vi "Transmitter.vi"() -> ()   [LabVIEW 2022 SP3]
uses:
  Transmitter States.ctl
  <vilib>/MakerHub/LINX/Public/Peripherals/Digital/Digital Write 1 Chan.vi
  <vilib>/MakerHub/LINX/Public/Peripherals/Digital/Digital Write N Chans.vi
  <vilib>/MakerHub/LINX/Private/Local IO/LinxDigitalWrite.vi
  <vilib>/MakerHub/LINX/Public/Utilities/Check Channel.vi
  <vilib>/MakerHub/LINX/Public/Utilities/Open Serial.vi
  <vilib>/MakerHub/LINX/Private/Utilties/Generate Error.vi
  <vilib>/MakerHub/LINX/LMH-LINX.lvlib
panel:
  out "Message Translated to Morse":string
  in  "stop":bool
  in  "Send Morse":bool
  in  "Message to Encode":string
  in  "Pulse Interval (ms)":u32=100
  in  "Serial Port":refnum<visa-resource-name>="N/A"
  in  "LED Channel":u8
  out "Message Transmitted":bool
  out "Digital Write Out":errorcluster
  out "File IO Error":errorcluster
  # "Morse Code Transmitter"
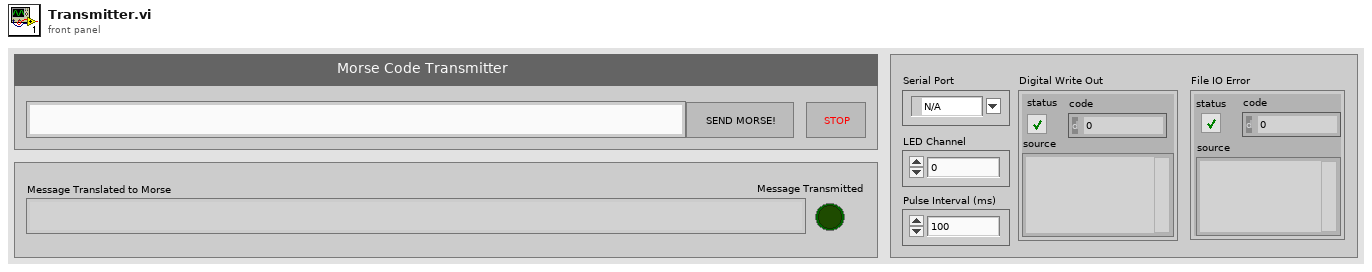
[diagram p1: front panel]
types:
  T1 = enum8{"Enabled", "Disabled", "Disabled and Grayed Out"}
  T2 = typedef "Transmitter States.ctl" = enum16{"Waiting for button press", "Button is pressed"}
  T3 = typedef "LMH-LINX.lvlib/LINX Ref.ctl" = cluster{"IO":T4, "Interface":T5, "LINX Device Config":T6}
  T4 = typedef "LMH-LINX.lvlib/Platform.ctl" = enum16{"Remote", "Local"}
  T5 = typedef "LMH-LINX.lvlib/Interface.ctl" = enum16{"Serial", "TCP"}
  T6 = typedef "LMH-LINX.lvlib/Device.lvlib/LINX Device Config.ctl" = cluster{"Interface":T5, "COM Port":refnum<visa-resource-name>, "TCP Configuration":T7, "Device Family":u8, "Device ID":u8, "Device Name":string, "TCP Ref":refnum<k5>, "Channels":T8}
  T7 = typedef "LMH-LINX.lvlib/Device.lvlib/TCP Config.ctl" = cluster{"IP Address":string, "Port":u16}
  T8 = typedef "LMH-LINX.lvlib/Channels.ctl" = cluster{"DI":u8[], "DO":u8[], "AI":u8[], "AO":u8[], "PWM":u8[], "QE":u8[], "UART":u8[], "I2C 2":u8[], "SPI":u8[], "CAN":u8[], "Servo":u8[], "AI Ref (V)":dbl, "AI Resolution (Bits)":u8, "AO Ref (V)":dbl, "AO Resolution (Bits)":u8}
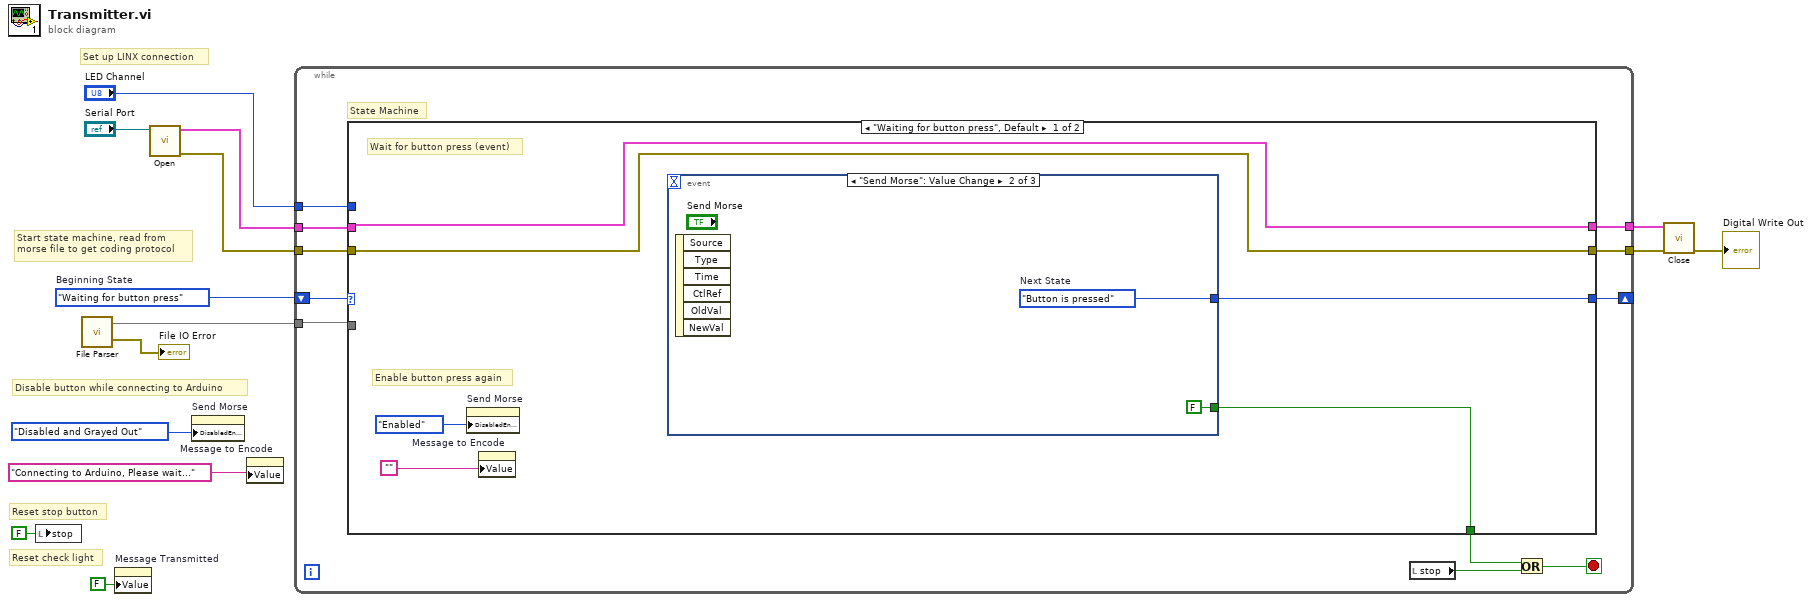
[diagram p0: block diagram]
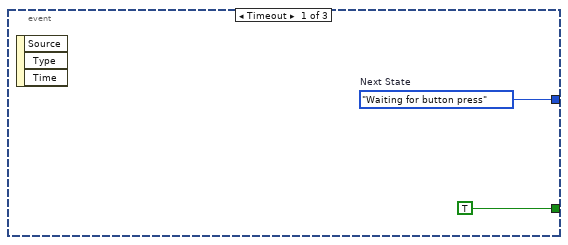
[diagram p2: hidden frame]
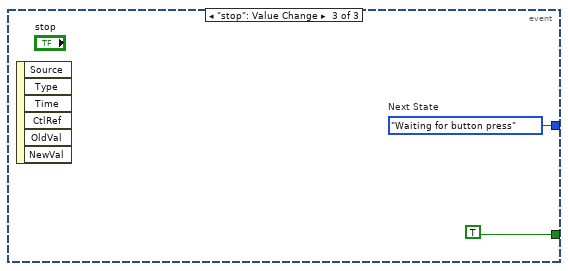
[diagram p3: hidden frame]
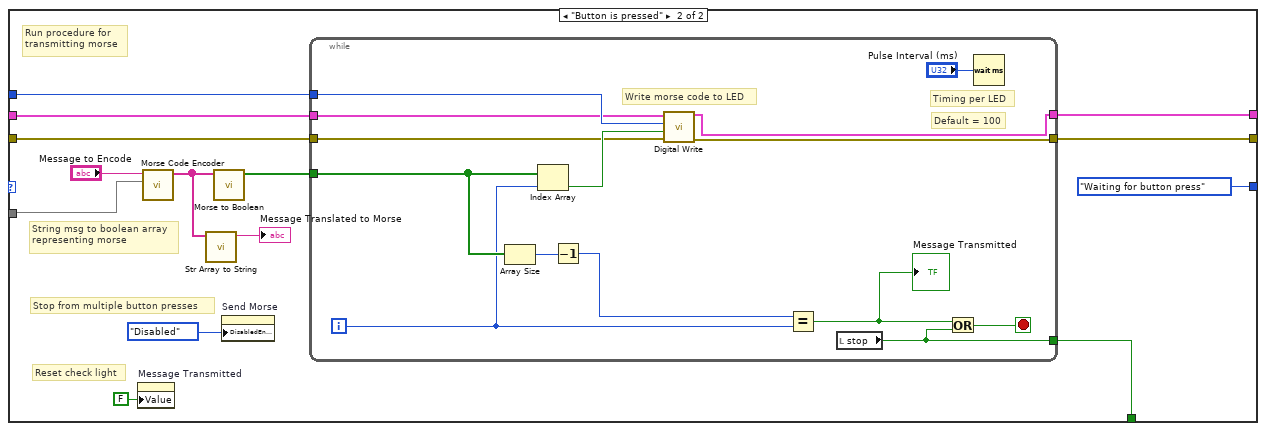
[diagram p4: hidden frame]
diagram:
  w12 = Transmitter_States."Waiting for button press"  # Beginning State
  # "Reset check light"
  # "Disable button while connecting to Arduino"
  # "Set up LINX connection"
  # "Reset stop button"
  # "Start state machine, read from\nmorse file to get coding protocol"
  n1 = local write "stop"(FALSE ("stop")) -> ()
  n2 = call "File Parser.vi"() -> ("error out"=→"File IO Error":errorcluster, "Letter-Morse Map (output 1)"=w13:map{string, string})  [unwired: 9 in, 1 out]
  n3 = property on="Message Transmitted" class="Bool (strict)"("Value"=FALSE ("Message Transmitted")) -> ()  [unwired: 2 in, 2 out]
  n4 = call-poly <vilib>:"Open.vi"("Serial Port"="Serial Port") -> ("Error Out"=w8:errorcluster, "LINX Resource"=w7:T3)  [unwired: 8 in, 1 out]
  n5 = property on="Send Morse" class="Bool"("DisabledEnum"=T1."Disabled and Grayed Out" ("Disabled")) -> ()  [unwired: 2 in, 2 out]
  n6 = property on="Message to Encode" class="Str"("Value"="Connecting to Arduino, Please wait..." ("Message Translated to Morse")) -> ()  [unwired: 2 in, 2 out]
  n7 = while {
    tunnel: w13 -> [w24]
    shift-right: [w25] -> _
    shift-left: w12 -> [w23]
    tunnel: "LED Channel" -> [w19]
    tunnel: w8 -> [w18]
    tunnel: w7 -> [w17]
    tunnel: [w16] -> w3
    tunnel: [w15] -> w1
    stop <- w22 stop-if-true
    # "State Machine"
    n8 = case shown="\"Waiting for button press\", Default" w23 {
      tunnel: w24 -> [_ w49]
      tunnel: [w31 Transmitter_States."Waiting for button press"] -> w25
      tunnel: [w30 w45] -> w21
      tunnel: w19 -> [_ w43]
      tunnel: w18 -> [w29 w42]
      tunnel: w17 -> [w26 w41]
      tunnel: [w29 w40] -> w16
      tunnel: [w26 w38] -> w15
      frame "Waiting for button press", Default {
        # "Enable button press again"
        # "Wait for button press (event)"
        n9 = property on="Send Morse" class="Bool"("DisabledEnum"=T1."Enabled" ("Disabled")) -> ()  [unwired: 2 in, 2 out]
        n10 = property on="Message to Encode" class="Str"("Value"="" ("Message Translated to Morse")) -> ()  [unwired: 2 in, 2 out]
        n11 = event shown="[1] \"Send Morse\": Value Change" {
          selector: _ -> [_ _ _]
          dyn-events: _ -> [_ _ _]
          timeout: _ -> [_ _ _]
          tunnel: [w33 w35 w36] -> w31
          tunnel: [TRUE ("stop") FALSE ("stop") TRUE ("stop")] -> w30
          event Timeout {
            w33 = Transmitter_States."Waiting for button press"  # Next State
            n12 = event-data() -> ()  [unwired: 1 in, 3 out]
          }
          event "Send Morse": Value Change {
            w35 = Transmitter_States."Button is pressed"  # Next State
            n13 = event-data() -> ()  [unwired: 1 in, 6 out]
          }
          event "stop": Value Change {
            w36 = Transmitter_States."Waiting for button press"  # Next State
            n14 = event-data() -> ()  [unwired: 1 in, 6 out]
          }
        }
      }
      frame "Button is pressed" {
        # "Reset check light"
        # "Stop from multiple button presses"
        # "Run procedure for\ntransmitting morse"
        # "String msg to boolean array representing morse"
        n15 = property on="Message Transmitted" class="Bool (strict)"("Value"=FALSE ("Message Transmitted")) -> ()  [unwired: 2 in, 2 out]
        n16 = call "Morse Code Encoder.vi"("Map"=w49, "Message to Encode"="Message to Encode") -> ("string array"=w47:string[])  [unwired: 9 in]
        n17 = call "Str Array to String.vi"("Array"=w47) -> ("String"=→"Message Translated to Morse":string)  [unwired: 10 in]
        n18 = call "Morse to Boolean.vi"("Morse Code Array"=w47) -> ("Boolean Array"=w50:bool[])  [unwired: 10 in]
        n19 = property on="Send Morse" class="Bool"("DisabledEnum"=T1."Disabled" ("Disabled")) -> ()  [unwired: 2 in, 2 out]
        n20 = while {
          tunnel: [w65] -> w40
          tunnel: w50 -> [w64]
          tunnel: w43 -> [w59]
          tunnel: [w55] -> w45
          tunnel: w42 -> [w54]
          tunnel: w41 -> [w53]
          tunnel: [w52] -> w38
          i -> [w61]
          stop <- w57 stop-if-true
          # "Default = 100"
          # "Timing per LED"
          # "Write morse code to LED"
          n21 = Array Size(array=w64) -> (size(s)=w63:i32)
          n22 = Index Array(array=w64, index=w61) -> (element=w60:bool)
          n23 = Decrement(x=w63) -> (x-1=w62:i32)
          n24 = call-poly <vilib>:"Digital Write.vi"("Error In"=w54, "Output Value"=w60, "DO Channel"=w59, "LINX Resource"=w53) -> ("Error Out"=w65:errorcluster, "LINX Resource"=w52:T3)  [unwired: 6 in]
          n25 = Equal?(x=w62, y=w61) -> (x = y?=w56:bool)
          "Message Transmitted" <- w56
          n26 = local read "stop"() -> (w55:bool)
          n27 = Or(x=w56, y=w55) -> (x .or. y?=w57:bool)
          n28 = Wait (ms)(milliseconds to wait="Pulse Interval (ms)") -> ()  [unwired: 1 out]
        }
      }
    }
    n29 = local read "stop"() -> (w20:bool)
    n30 = Or(x=w21, y=w20) -> (x .or. y?=w22:bool)
  }
  n31 = call <vilib>:"Close.vi"("Error In"=w3, "LINX Resource"=w1) -> ("Error Out"=→"Digital Write Out":errorcluster)  [unwired: 9 in]
